vi "ReadXLSConfig.vi"(8 "error in (no error)":errorcluster caption="错误输入（无错误）", 10 "产品型号":refnum<vi>, 11 "XLSName":string) -> (0 "error out":errorcluster, 3 "Data":string[][](array[string]))   [LabVIEW 2013]
uses:
  <vilib>/Utility/NIReport.llb/NI_report.lvclass
  GlobalValue.vi
  <vilib>/addons/_office/excel.llb/Excel Get Data ([str]).vi
  <vilib>/addons/_office/NI_ReportGenerationToolkit.lvlib
  <vilib>/Utility/NIReport.llb/Excel/NI_Excel.lvclass
panel:
  out "已删除的部分":string[](array[string])
  out "ConfigPath":string="C:\\Users\\dell\\Desktop\\ExcelReport.vi"
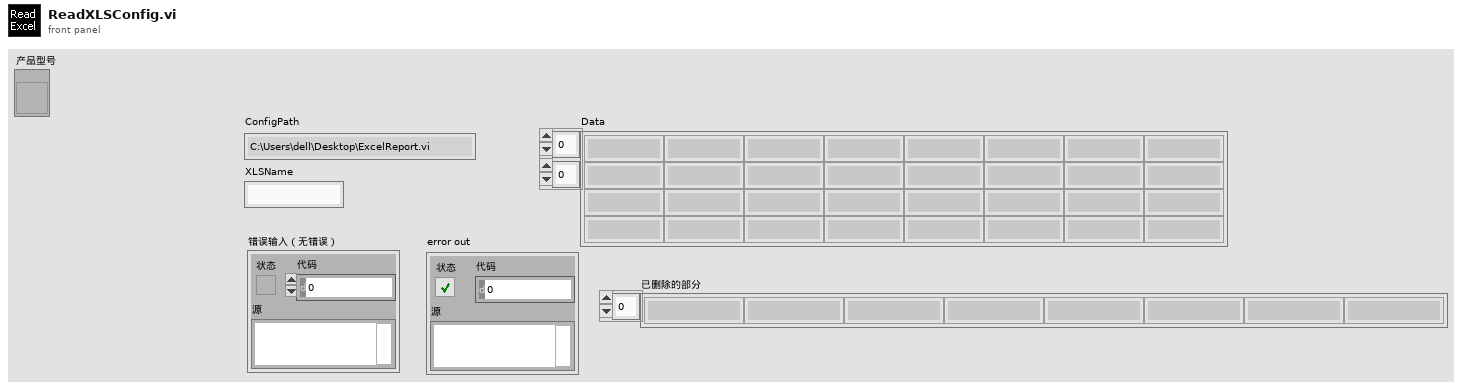
[diagram p1: front panel]
types:
  T1 = enum16{"maximized", "minimized", "normal", "no change"}
  T2 = enum16{"Standard Report", "HTML", "Word", "Excel"}
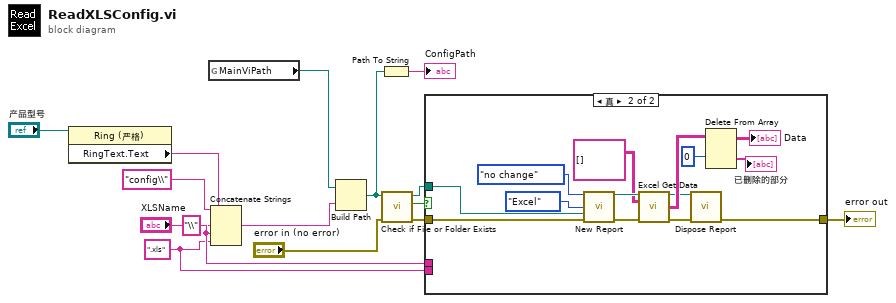
[diagram p0: block diagram]
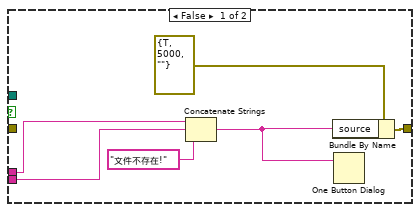
[diagram p2: hidden frame]
diagram:
  w6 = ".xls" ("字符串")
  n1 = property on="属性节点" class="Ring (严格)"(reference="产品型号") -> ("RingText.Text"=w3:string)  [unwired: 1 in, 2 out]
  n2 = global read "GlobalValue.vi" "MainViPath"() -> (w5:path)
  n3 = Concatenate Strings("config\\" ("连接的字符串"), w3, "\\" ("字符串"), "XLSName", w6) -> (w8:string)
  n4 = Build Path(base path=w5, name or relative path=w8) -> (appended path=w14:path)
  n5 = Path To String(path=w14) -> (string=→"ConfigPath":string)
  n6 = call <vilib>:"Check if File or Folder Exists.vi"("error in (no error)"="error in (no error)", "path"=w14) -> ("error out"=w12:errorcluster, "file or folder exists?"=w13:bool, "dup path"=w11:path)  [unwired: 7 out]
  n7 = case shown="真" w13 {
    tunnel: w11 -> [_ w26]
    tunnel: [w21 w25] -> w10
    tunnel: w12 -> [_ w24]
    tunnel: "XLSName" -> [w20 _]
    tunnel: w6 -> [w19 _]
    frame False {
      n8 = Concatenate Strings(w20, w19, "文件不存在!" ("消息")) -> (w17:string)
      n9 = Bundle By Name(cluster=errorcluster {"status"=TRUE, "code"=5000, "source"=""} ("error in 1 (no error)"), "source"=w17) -> (w21:errorcluster)
      n10 = One Button Dialog(message=w17) -> ()  [unwired: 1 in, 1 out]
    }
    frame True {
      n11 = call <vilib>:"New Report.vi"("window state (normal)"=T1."no change", "report type"=T2."Excel", "template (empty)"=w26, "error in (no error)"=w24) -> ("report out"=w31:refnum<class "NI_report.lvclass">, "error out"=w32:errorcluster)  [unwired: 2 in, 8 out]
      n12 = call-poly <vilib>:"Excel Get Data.vi"("report in"=w31, "data type"=string[][] [], "error in (no error)"=w32) -> ("report out"=w28:refnum<class "NI_report.lvclass">, "data"=w33:string[][], "error out"=w27:errorcluster)  [unwired: 10 in]
      n13 = call-dynamic "Dispose Report.vi"("report in"=w28, "error in (no error)"=w27) -> ("error out"=w25:errorcluster)  [unwired: 3 in, 10 out]
      n14 = Delete From Array(array=w33, index (row)=0 ("索引 (行)")) -> (deleted portion=→"已删除的部分":string[], array with subset deleted=→"Data":string[][])  [unwired: 2 in]
    }
  }
  "error out" <- w10
